vi "En_Disen_output.vi"(8 "error in (no error)":errorcluster, 10 "newstate":bool, 11 "Connection":T1={"Baud"=9600, "Flow Ctl"=0, "COM port"="", "Parity"=0} {"Parity" items=["None", "Odd", "Even"]; "Flow Ctl" items=["None"]; "Baud" items=["4800"=4800, "9600"=9600, "19200"=19200, "38400"=38400]}) -> (0 "error out":errorcluster, 2 "actual_state":bool, 3 "Connection out":T1={"Baud"=9600, "Flow Ctl"=0, "COM port"="", "Parity"=0} {"Parity" items=["None", "Odd", "Even"]; "Flow Ctl" items=["None"]; "Baud" items=["4800"=4800, "9600"=9600, "19200"=19200, "38400"=38400]})   [LabVIEW 2014, in "B&K Precision 9120 series.lvclass"]
uses:
  B&K Precision 9120 series.lvclass
  Serial_Config.ctl
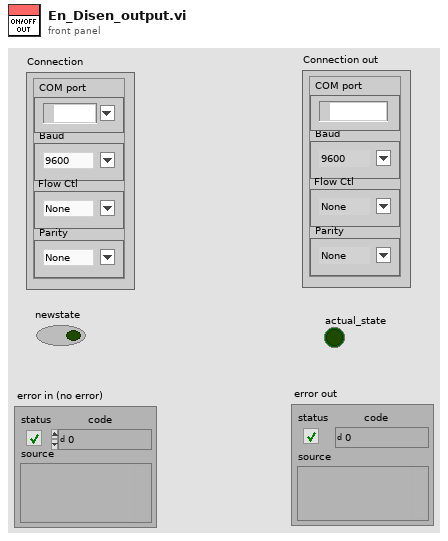
[diagram p1: front panel]
types:
  T1 = typedef "B&K Precision 9120 series.lvclass/Serial_Config.ctl" = cluster{"Baud":u32, "Flow Ctl":u16, "COM port":refnum<visa-resource-name>, "Parity":u16}
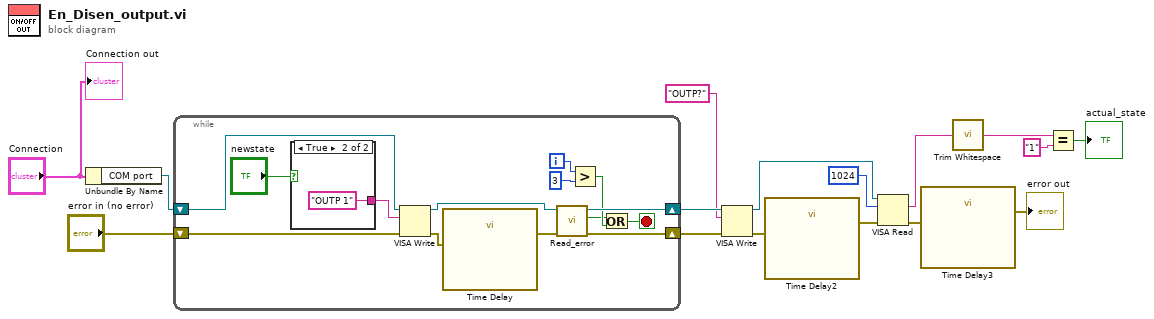
[diagram p0: block diagram]
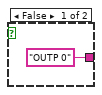
[diagram p2: hidden frame]
diagram:
  n1 = Unbundle By Name("Connection") -> ("COM port"=w6:refnum<visa-resource-name>)
  n2 = while {
    shift-right: [w27] -> w15
    shift-left: w6 -> [w30]
    shift-right: [w26] -> w13
    shift-left: "error in (no error)" -> [w29]
    i -> [w22]
    stop <- w23 stop-if-true
    n3 = case shown="True" "newstate" {
      tunnel: ["OUTP 0" ("write buffer") "OUTP 1" ("write buffer")] -> w20
      frame False {
      }
      frame True {
      }
    }
    n4 = VISA Write(VISA resource name=w30, write buffer=w20, error in (no error)=w29) -> (VISA resource name out=w28:refnum<visa-resource-name>, error out=w18:errorcluster)  [unwired: 1 out]
    n5 = call "Time Delay"("error in (no error)"=w18) -> ("error out"=w17:errorcluster)  [unwired: 10 in]
    n6 = call "Read_error.vi"("error in (no error)"=w17, "VISA resource in"=w28) -> ("error out"=w26:errorcluster, "OK"=w21:bool, "VISA resource out"=w27:refnum<visa-resource-name>)  [unwired: 7 in]
    n7 = Greater?(x=w22, y=3) -> (0:w25:bool)
    n8 = Or(x=w21, y=w25) -> (x .or. y?=w23:bool)
  }
  n9 = VISA Write(VISA resource name=w15, write buffer="OUTP?", error in (no error)=w13) -> (VISA resource name out=w12:refnum<visa-resource-name>, error out=w4:errorcluster)  [unwired: 1 out]
  n10 = call "Time Delay2"("error in (no error)"=w4) -> ("error out"=w3:errorcluster)  [unwired: 10 in]
  n11 = VISA Read(VISA resource name=w12, byte count=u32 1024, error in (no error)=w3) -> (read buffer=w10:string, error out=w2:errorcluster)  [unwired: 2 out]
  n12 = call "Time Delay3"("error in (no error)"=w2) -> ("error out"=→"error out":errorcluster)  [unwired: 10 in]
  n13 = call <vilib>:"Trim Whitespace.vi"("string"=w10) -> ("trimmed string"=w8:string)  [unwired: 1 in]
  n14 = Equal?(x=w8, y="1") -> (x = y?=→"actual_state":bool)
  "Connection out" <- "Connection"
